vi "main2.vi"() -> ()   [LabVIEW 2009]
uses:
  <vilib>/Instr/_visa.llb/VISA Configure Serial Port (Instr).vi
panel:
  in  "停止":bool
  in  "delay before read (ms)":u32=500 caption="读取前延时(ms)"
  in  "flow control":u16(ring) caption="流程控制" items=["无"=0, "XON/XOFF"=1, "RTS/CTS"=2, "DTR/DSR"=4]
  in  "stop bits":u16(ring)=10 caption="停止位" items=["1.0"=10, "1.5"=15, "2.0"=20]
  in  "parity":u16(ring) caption="奇偶" items=["无", "奇", "偶", "标记", "空格"]
  in  "data bits":u16=8 caption="数据比特" min=5 max=8 step=1
  out "read string":string caption="读取字符串"
  in  "VISA resource name":refnum<visa-resource-name>="COM1" caption="VISA资源名称"
  in  "baud rate":u32=9600 caption="波特率"
  in  "Spoken Text":string
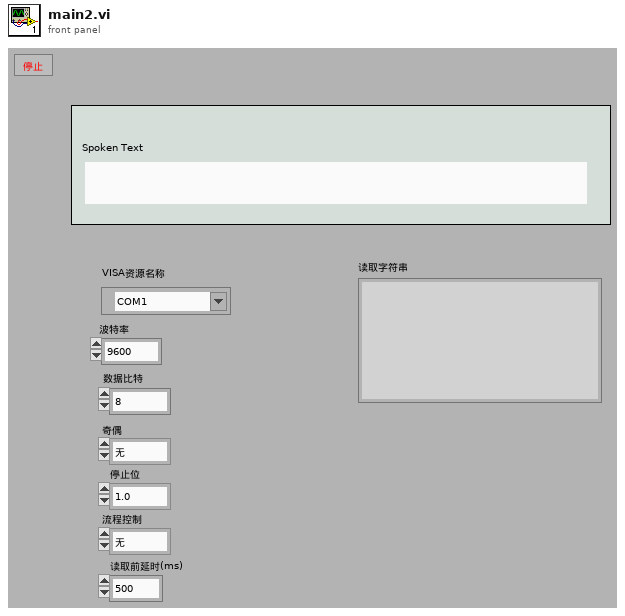
[diagram p1: front panel]
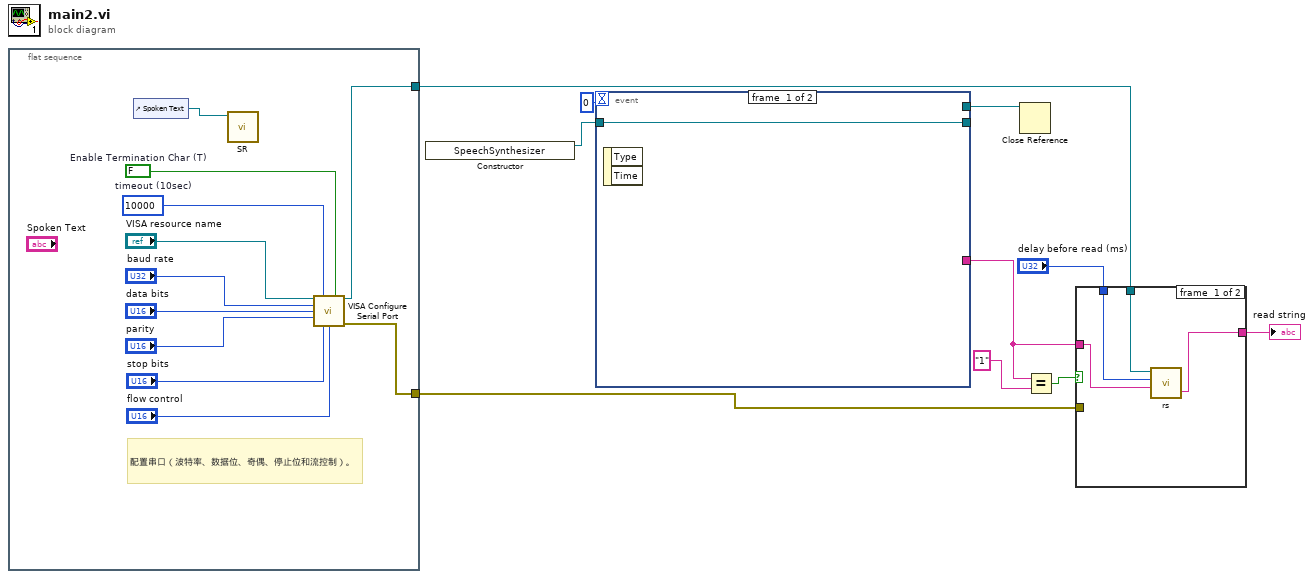
[diagram p0: block diagram]
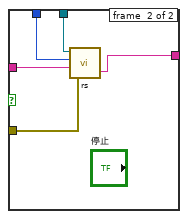
[diagram p2: hidden frame]
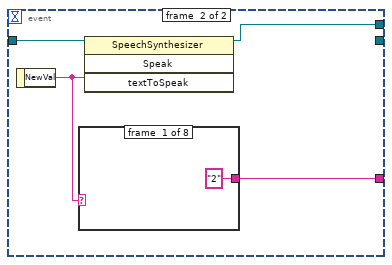
[diagram p3: hidden frame]
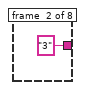
[diagram p4: hidden frame]
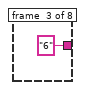
[diagram p5: hidden frame]
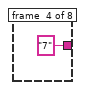
[diagram p6: hidden frame]
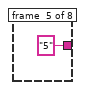
[diagram p7: hidden frame]
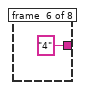
[diagram p8: hidden frame]
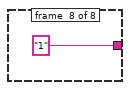
[diagram p10: hidden frame]
diagram:
  n1 = flat-sequence {
    tunnel: [w21] -> w7
    tunnel: [w20] -> w6
    frame #0 {
      w14 = FALSE  # Enable Termination Char (T)
      w15 = u32 10000  # timeout (10sec)
      # "配置串口（波特率、数据位、奇偶、停止位和流控制）。"
      n2 = control-ref of="Spoken Text"() -> (w19:refnum<vi>)
      n3 = call "SR.vi"("Spoken text box"=w19) -> ()  [unwired: 6 in, 1 out]
      n4 = call-poly "VISA Configure Serial Port"("VISA resource name"="VISA resource name", "timeout (10sec)"=w15, "Enable Termination\nChar (T)"=w14, "baud rate (9600)"="baud rate", "data bits (8)"="data bits", "parity (0:none)"="parity", "stop bits (10: 1 bit)"="stop bits", "flow control (0:none)"="flow control") -> ("VISA resource name out"=w20:refnum<visa-resource-name>, "error out"=w21:errorcluster)  [unwired: 1 in, 5 out]
    }
  }
  n5 = constructor class="SpeechSynthesizer"() -> (reference out=w10:refnum<k24>)  [unwired: 3 in, 2 out]
  n6 = event shown="[1] \"Spoken Text\": 值改变" {
    selector: _ -> [_ _]
    dyn-events: _ -> [_ _]
    timeout: 0 -> [_ _]
    tunnel: w10 -> [w22 w26]
    tunnel: [w22 _] -> _
    tunnel: [_ w24] -> w9
    tunnel: [_ w23] -> w1
    event #0 {
      n7 = event-data() -> ()  [unwired: 1 in, 2 out]
    }
    event #1 {
      n8 = event-data() -> ("NewVal"=w25:string)  [unwired: 1 in]
      n9 = case shown="\"前进\"" w25 {
        tunnel: ["2" "3" "6" "7" "5" "4" _ "1"] -> w23
        frame #0 {
        }
        frame #1 {
        }
        frame #2 {
        }
        frame #3 {
        }
        frame #4 {
        }
        frame #5 {
        }
        frame #6 {
        }
        frame #7 {
        }
      }
      n10 = invoke class="SpeechSynthesizer" method="Speak"(reference=w26, "textToSpeak"=w25) -> (reference out=w24:refnum<k24>)  [unwired: 2 in, 3 out]
    }
  }
  n11 = Close Reference(reference=w9) -> ()  [unwired: 1 in, 1 out]
  n12 = Equal?(x=w1, y="1") -> (x = y?=w2:bool)
  n13 = case shown="真" w2 {
    tunnel: w7 -> [_ w42]
    tunnel: w6 -> [w37 w41]
    tunnel: "delay before read (ms)" -> [w36 w40]
    tunnel: [w35 w39] -> w3
    tunnel: w1 -> [w34 w38]
    frame #0 {
      n14 = call "rs.vi"("字符串"=w34, "delay before read (ms)"=w36, "VISA resource name out"=w37) -> ("read string"=w35:string)  [unwired: 2 in]
    }
    frame #1 {
      n15 = call "rs.vi"("error out"=w42, "字符串"=w38, "delay before read (ms)"=w40, "VISA resource name out"=w41) -> ("read string"=w39:string)  [unwired: 1 in]
    }
  }
  "read string" <- w3
